vi "Timer.vi"(10 "Timer Control":T1=enum."Start", 11 "Time Target":dbl format="%0.2f") -> (2 "Time completed?":bool=TRUE, 3 "Elapsed Time":dbl format="%0.2f")   [LabVIEW 2020]
doc: "Timer with Star, Stop and Reset functions."
uses:
  Controls/Timer Controls.ctl
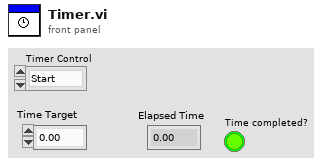
[diagram p1: front panel]
types:
  T1 = typedef "Timer Controls.ctl" = enum16{"Reset", "Start", "Stop"}
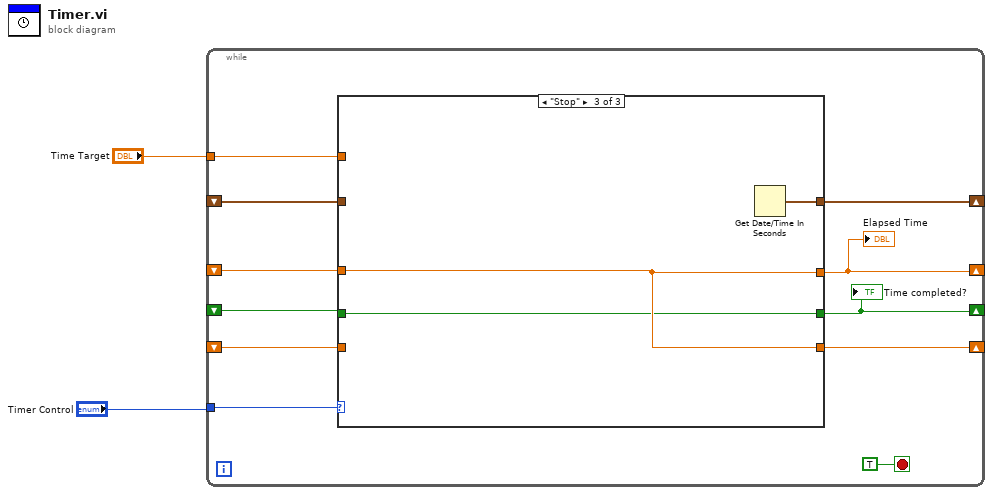
[diagram p0: block diagram]
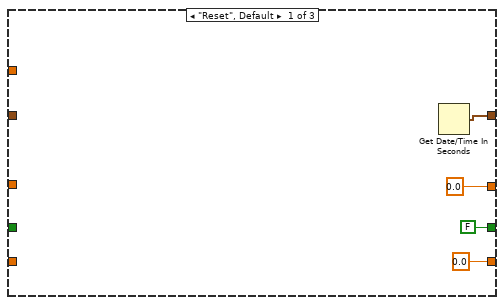
[diagram p2: hidden frame]
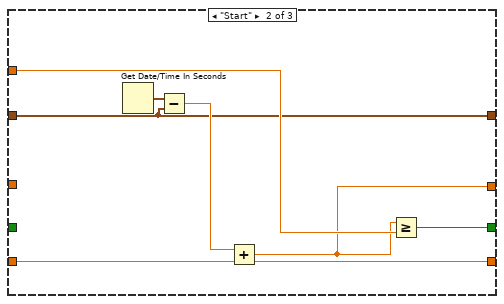
[diagram p3: hidden frame]
diagram:
  n1 = while {
    tunnel: "Time Target" -> [w12]
    tunnel: "Timer Control" -> [w11]
    shift-right: [w10] -> _
    shift-left: _ -> [w9]
    shift-right: [w8] -> _
    shift-left: _ -> [w7]
    shift-right: [w6] -> _
    shift-left: _ -> [w5]
    shift-right: [w4] -> _
    shift-left: _ -> [w3]
    stop <- TRUE stop-if-true
    n2 = case shown="\"Stop\"" w11 {
      tunnel: [0.0 ("Elapsed Time 2") w19 w26] -> w6
      tunnel: w12 -> [_ w23 _]
      tunnel: [FALSE ("Boolean") w22 w25] -> w4
      tunnel: [w15 w18 w27] -> w10
      tunnel: w9 -> [_ w18 _]
      tunnel: [0.0 ("Elapsed Time 2") w20 w26] -> w8
      tunnel: w7 -> [_ w20 _]
      tunnel: w5 -> [_ _ w26]
      tunnel: w3 -> [_ _ w25]
      frame "Reset", Default {
        n3 = Get Date/Time In Seconds() -> (seconds since 1Jan1904=w15:timestamp)
      }
      frame "Start" {
        n4 = Get Date/Time In Seconds() -> (seconds since 1Jan1904=w24:timestamp)
        n5 = Subtract(x=w24, y=w18) -> (x-y=w21:dbl)
        n6 = Add(x=w21, y=w20) -> (x+y=w19:dbl)
        n7 = Greater Or Equal?(x=w19, y=w23) -> (x >= y?=w22:bool)
      }
      frame "Stop" {
        n8 = Get Date/Time In Seconds() -> (seconds since 1Jan1904=w27:timestamp)
      }
    }
    "Elapsed Time" <- w6
    "Time completed?" <- w4
  }
